vi "Calculate rotation amount based on orientation.vi"(0 "Orientation":dbl, 1 "Desired orientation":dbl, 5 "Min orientation for rotation":dbl=3.0, 7 "Orientation for max rotation":dbl=30.0, 9 "Rot min abs spd":dbl=0.5, 11 "error in":errorcluster, 12 "Rot spd multiplier":dbl=5.0) -> (4 "Rot spd percentage (0 to 1)":dbl, 6 "angle needed to rotate":dbl, 14 "Rot spd out":dbl, 15 "error out":errorcluster)   [LabVIEW 2017]
uses:
  <vilib>/Analysis/coordinate.llb/Angle Range (Degree).ctl
  <vilib>/Analysis/coordinate.llb/Angle Units.ctl
  <vilib>/Analysis/coordinate.llb/Wrap Angle (scalar).vi
  <vilib>/Analysis/NI_AAL_Angle.lvlib
panel:
  out "Raw rot speed out":dbl
  # "VI Description: Calculates the desired rotational speed of the motors to correct orientation.\nPositive rotational speed = clockwise"
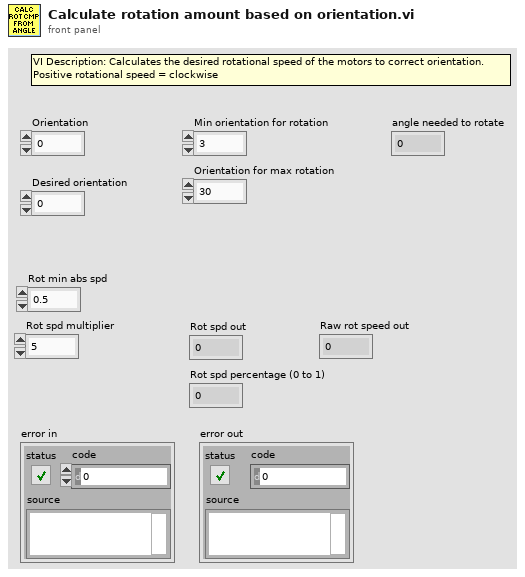
[diagram p1: front panel]
types:
  T1 = typedef "NI_AAL_Angle.lvlib/Angle Units.ctl" = i32
  T2 = typedef "NI_AAL_Angle.lvlib/Angle Range (Degree).ctl" = u16
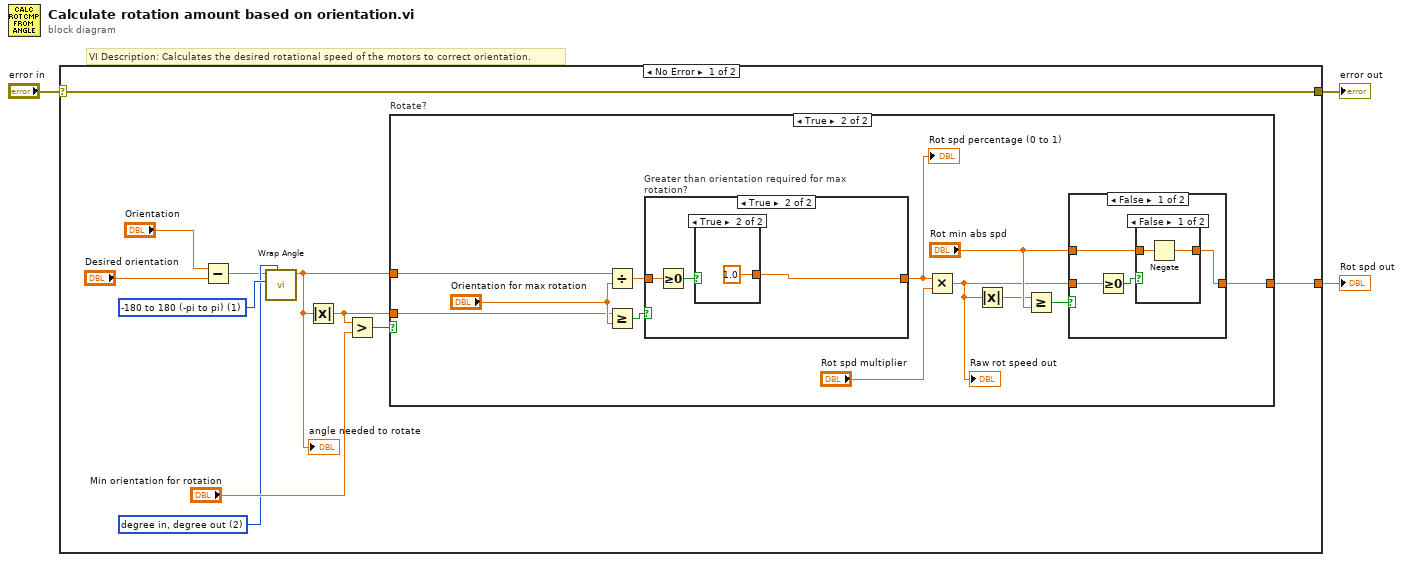
[diagram p0: block diagram]
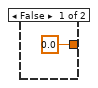
[diagram p2: hidden frame]
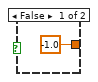
[diagram p6: hidden frame]
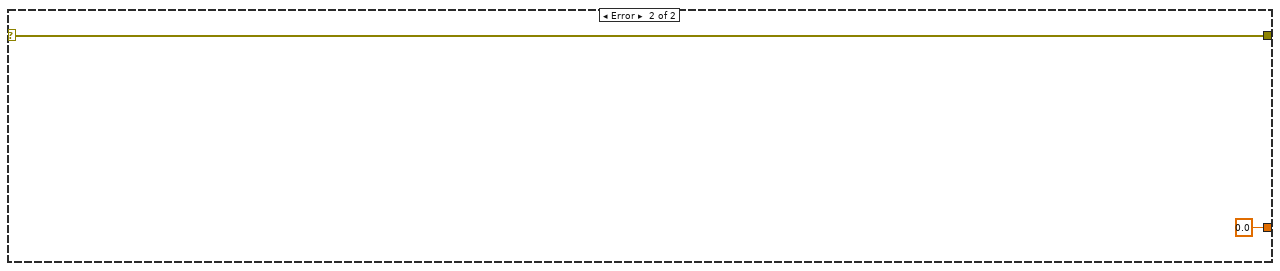
[diagram p7: hidden frame]
diagram:
  # "VI Description: Calculates the desired rotational speed of the motors to correct orientation."
  n1 = case shown="No Error" "error in" {
    selector: "error in" -> [w12 w43]
    tunnel: [w12 w43] -> w2
    tunnel: [w11 0.0 ("Min absolute speed")] -> w1
    frame No Error {
      w6 = T1 2 items=["radian in, radian out", "radian in, degree out", "degree in, degree out", "degree in, radian out"] ("angle units")
      w7 = T2 1 items=["none", "-180 to 180 (-pi to pi)", "0 to 360 (0 to 2pi)"] ("angle range")
      n2 = Subtract(x="Orientation", y="Desired orientation") -> (x-y=w5:dbl)
      n3 = call-poly <vilib>:"Wrap Angle.vi"("angle units"=w6, "angle range"=w7, "angle in"=w5) -> ("angle out"=w4:dbl)  [unwired: 7 in, 1 out]
      "angle needed to rotate" <- w4
      n4 = Absolute Value(x=w4) -> (abs(x)=w10:dbl)
      n5 = Greater?(x=w10, y="Min orientation for rotation") -> (0:w13:bool)
      n6 = case "Rotate?" shown="True" w13 {
        tunnel: w4 -> [_ w18]
        tunnel: [0.0 ("Min absolute speed") w20] -> w11
        tunnel: w10 -> [_ w19]
        frame False {
        }
        frame True {
          n7 = Divide(x=w18, y="Orientation for max rotation") -> (x/y=w25:dbl)
          n8 = Greater Or Equal?(x=w19, y="Orientation for max rotation") -> (x >= y?=w26:bool)
          n9 = case "Greater than orientation required for max rotation?" shown="True" w26 {
            tunnel: [w36 w38] -> w23
            tunnel: w25 -> [w36 w37]
            frame False {
            }
            frame True {
              n10 = Greater Or Equal To 0?(x=w37) -> (x >= 0?=w39:bool)
              n11 = case shown="True" w39 {
                tunnel: [-1.0 ("speed out") 1.0 ("speed out")] -> w38
                frame False {
                }
                frame True {
                }
              }
            }
          }
          "Rot spd percentage (0 to 1)" <- w23
          n12 = Multiply(x=w23, y="Rot spd multiplier") -> (x*y=w17:dbl)
          "Raw rot speed out" <- w17
          n13 = Absolute Value(x=w17) -> (abs(x)=w16:dbl)
          n14 = Greater Or Equal?(x=w16, y="Rot min abs spd") -> (x >= y?=w24:bool)
          n15 = case shown="False" w24 {
            tunnel: w17 -> [w30 w35]
            tunnel: [w28 w35] -> w20
            tunnel: "Rot min abs spd" -> [w29 _]
            frame False {
              n16 = Greater Or Equal To 0?(x=w30) -> (x >= 0?=w31:bool)
              n17 = case shown="False" w31 {
                tunnel: w29 -> [w33 w34]
                tunnel: [w32 w34] -> w28
                frame False {
                  n18 = Negate(x=w33) -> (-x=w32:dbl)
                }
                frame True {
                }
              }
            }
            frame True {
            }
          }
        }
      }
    }
    frame Error {
    }
  }
  "error out" <- w2
  "Rot spd out" <- w1
